vi "core_module.vi"(8 "error in (no error)":errorcluster) -> (0 "error out":errorcluster, 1 "modbusData":refnum<notifier>, 2 "Instrument out":refnum<class "Instrument.lvclass">, 3 "userEvent":T1, 5 "Cluster":T2)   [LabVIEW 2019]
uses:
  instrument/Instrument.lvclass
  core_dataRefCluster.ctl
  core_dataRef.ctl
  core_dataCluster.ctl
  instrument/instr_dataCluster.ctl
  gui/ecu_dataCluster.ctl
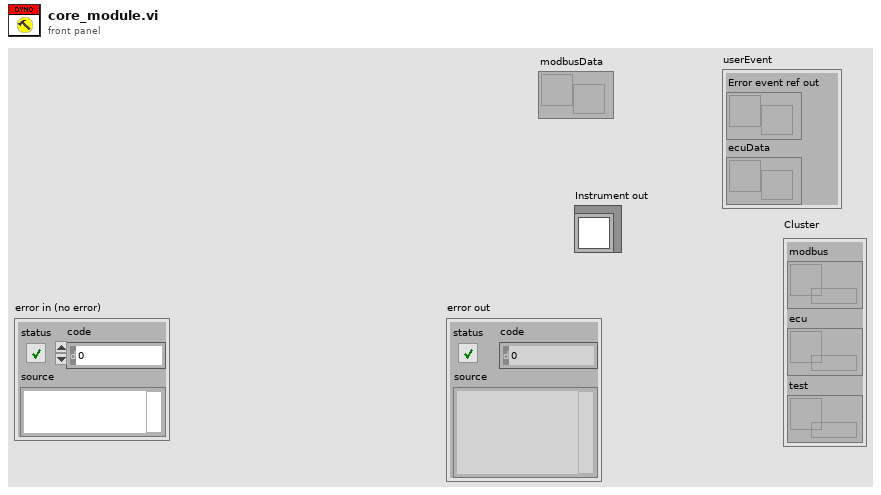
[diagram p1: front panel]
types:
  T1 = cluster{"Error event ref out":refnum<user-event>, "ecuData":refnum<user-event>}
  T2 = typedef "core_dataRefCluster.ctl" = cluster{"modbus":T3, "ecu":T3, "test":T3}
  T3 = typedef "core_dataRef.ctl" = refnum<queue>
  T4 = enum16{"Initialize", "Check Error", "Report Error"}
  T5 = typedef "Instrument.lvclass/instr_dataCluster.ctl" = cluster{"电源电压 V":dbl, "电源电流A":dbl, "扭矩N/m":dbl, "速度r/M":dbl, "温度℃":dbl[], "流量计L/M":dbl[]}
  T6 = typedef "core_dataCluster.ctl" = cluster{"cmd":string, "data":variant}
  T7 = typedef "ecu_dataCluster.ctl" = cluster{"MCU_MotCtrlrSts":dbl, "MCU_MotTq":dbl, "MCU_MotBusU":dbl, "MCU_MotSpd":dbl, "MCU_MotBodyT":dbl, "MCU_MotBody_T":dbl, "MCU_MotCtrlrT":dbl, "MCU 状态":bool, "ErrMsg":i64}
  T8 = cluster{"Queue Ref out[0]":T3, "Queue Ref out[1]":T3, "Queue Ref out[2]":T3}
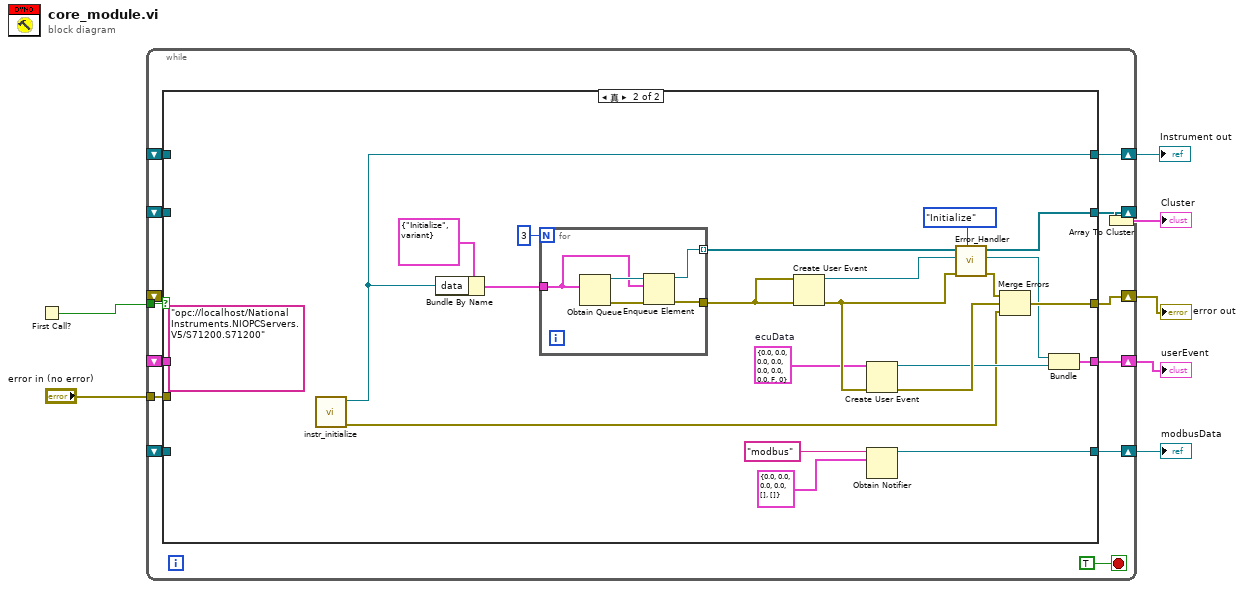
[diagram p0: block diagram]
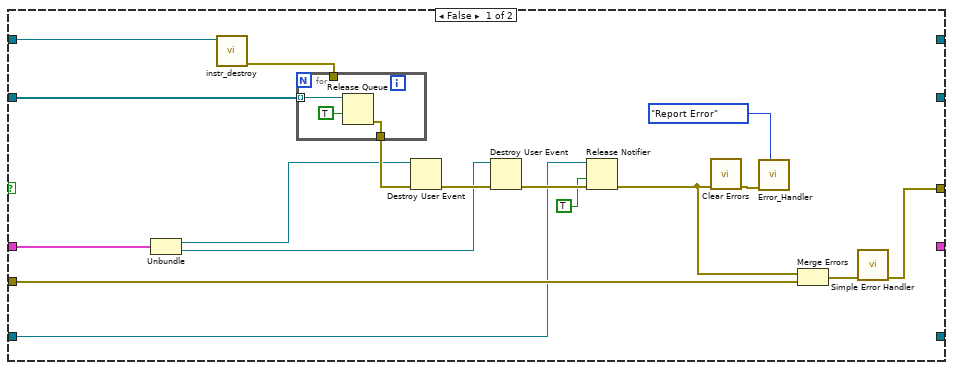
[diagram p2: hidden frame]
diagram:
  n1 = First Call?() -> (First Call?: T/F=w8:bool)
  n2 = while {
    tunnel: w8 -> [w20]
    shift-right: [w19] -> w5
    shift-left: _ -> [w18]
    shift-right: [w16] -> w2
    shift-left: _ -> [w13]
    shift-right: [w14] -> w3
    shift-left: _ -> [w12]
    tunnel: "error in (no error)" -> [w11]
    shift-right: [w10] -> w4
    shift-left: _ -> [w9]
    shift-right: [w15] -> w7
    shift-left: _ -> [_]
    stop <- TRUE stop-if-true
    n3 = case shown="真" w20 {
      tunnel: [_ w59] -> w19
      tunnel: w18 -> [w37 _]
      tunnel: [_ w54] -> w16
      tunnel: [w29 w51] -> w15
      tunnel: [_ w46] -> w14
      tunnel: w13 -> [w36 _]
      tunnel: w12 -> [w34 _]
      tunnel: w11 -> [w31 _]
      tunnel: [_ w43] -> w10
      tunnel: w9 -> [w24 _]
      frame False {
        n4 = Unbundle(w34) -> ("Error event ref out"=w26:refnum<user-event>, "ecuData"=w25:refnum<user-event>)
        n5 = call "instr_destroy.vi"("Instrument in"=w37) -> ("error out"=w35:errorcluster)  [unwired: 10 in]
        n6 = for {
          tunnel: w36 -> [w40] mode=indexing
          tunnel: w35 -> [_]
          tunnel: [w38] -> w33
          n7 = Release Queue(queue=w40, force destroy? (F)=TRUE) -> (error out=w38:errorcluster)  [unwired: 1 in, 2 out]
        }
        n8 = Destroy User Event(user event=w26, error in=w33) -> (error out=w28:errorcluster)
        n9 = Destroy User Event(user event=w25, error in=w28) -> (error out=w27:errorcluster)
        n10 = Release Notifier(notifier=w24, force destroy? (F)=TRUE, error in (no error)=w27) -> (error out=w21:errorcluster)  [unwired: 2 out]
        n11 = call <vilib>:"Clear Errors.vi"("error in (no error)"=w21) -> ("error out"=w22:errorcluster)  [unwired: 5 in, 1 out]
        n12 = call "Error_Handler.vi"("error mode"=T4."Report Error", "error in"=w22) -> ()  [unwired: 7 in, 3 out]
        n13 = Merge Errors(w21, w31) -> (w30:errorcluster)
        n14 = call <vilib>:"Simple Error Handler.vi"("error in (no error)"=w30) -> ("error out"=w29:errorcluster)  [unwired: 4 in, 4 out]
      }
      frame True {
        (unwired) "opc://localhost/National Instruments.NIOPCServers.V5/S71200.S71200" ("OPC Server")
        w41 = T7 {"MCU_MotCtrlrSts"=0.0, "MCU_MotTq"=0.0, "MCU_MotBusU"=0.0, "MCU_MotSpd"=0.0, "MCU_MotBodyT"=0.0, "MCU_MotBody_T"=0.0, "MCU_MotCtrlrT"=0.0, "MCU 状态"=FALSE, "ErrMsg"=0}  # ecuData
        n15 = call "instr_initialize.vi"() -> ("error out"=w42:errorcluster, "Instrument out"=w59:refnum<class "Instrument.lvclass">)  [unwired: 10 in]
        n16 = Bundle By Name(cluster=T6 {"cmd"="Initialize", "data"=variant} ("Cluster"), "data"=w59) -> (w60:T6)
        n17 = for {
          N: 3 -> [_]
          tunnel: w60 -> [w63]
          tunnel: [w62] -> w55 mode=indexing
          tunnel: [w65] -> w57
          n18 = Obtain Queue(element data type=w63) -> (queue out=w64:refnum<queue>, error out=w66:errorcluster)  [unwired: 4 in, 1 out]
          n19 = Enqueue Element(queue=w64, element=w63, error in (no error)=w66) -> (queue out=w62:refnum<queue>, error out=w65:errorcluster)  [unwired: 1 in, 1 out]
        }
        n20 = Create User Event(user event datatype=w57, error in=w57) -> (user event=w56:refnum<user-event>, error out=w49:errorcluster)
        n21 = Create User Event(user event datatype=w41, error in=w49) -> (user event=w48:refnum<user-event>, error out=w50:errorcluster)
        n22 = Obtain Notifier(name (unnamed)="modbus", notification data type=T5 {"电源电压 V"=0.0, "电源电流A"=0.0, "扭矩N/m"=0.0, "速度r/M"=0.0, "温度℃"=[], "流量计L/M"=[]} ("Cluster")) -> (notifier out=w43:refnum<notifier>)  [unwired: 2 in, 2 out]
        n23 = call "Error_Handler.vi"("error mode"=T4."Initialize", "error in"=w49, "Error event ref"=w56, "Queue Ref in"=w55) -> ("error out"=w52:errorcluster, "Error event ref out"=w47:refnum<user-event>, "Queue Ref out"=w54:T3[])  [unwired: 5 in]
        n24 = Merge Errors(w52, w50, w42) -> (w51:errorcluster)
        n25 = Bundle("Error event ref out"=w47, "ecuData"=w48) -> (w46:T1)  [unwired: 1 in]
      }
    }
  }
  "error out" <- w7
  "Instrument out" <- w5
  "modbusData" <- w4
  "userEvent" <- w3
  n26 = Array To Cluster(array=w2) -> (cluster=→"Cluster":T8)
